vi "Switch.vi"(6 "Command Info In":T1, 8 "Position":T4=enum."Far Right") -> (0 "Command Info Out":T1)   [LabVIEW 2017]
uses:
  Support Code/Starting Position.ctl
  <vilib>/Rock Robotics/WPI/Framework/Command Status Info.ctl
  <vilib>/Rock Robotics/WPI/Framework/Completion Status.ctl
  <vilib>/Rock Robotics/WPI/Framework/Completion Notifier.ctl
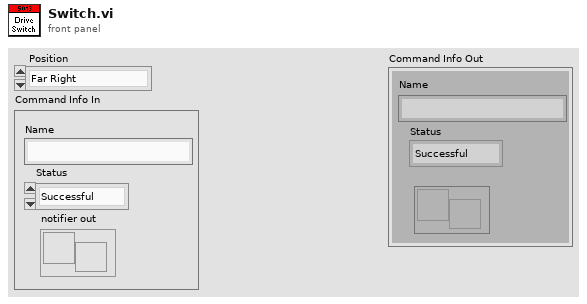
[diagram p1: front panel]
types:
  T1 = typedef "Command Status Info.ctl" = cluster{"Name":string, "Status":T2, "notifier out":T3}
  T2 = typedef "Completion Status.ctl" = enum16{"Successful", "Aborted", "Incomplete"}
  T3 = typedef "Completion Notifier.ctl" = refnum<notifier>
  T4 = typedef "Starting Position.ctl" = enum16{"Far Left", "Center", "Far Right"}
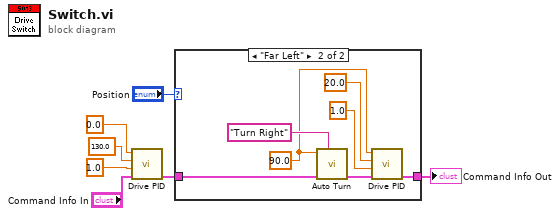
[diagram p0: block diagram]
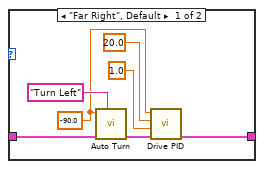
[diagram p2: hidden frame]
diagram:
  n1 = call "Drive PID.vi"("Command Info In"="Command Info In", "Speed"=1.0, "Distance"=130.0, "Target Angle"=0.0 ("Distance")) -> ("Command Info Out"=w5:T1)  [unwired: 7 in]
  n2 = case shown="\"Far Left\"" "Position" {
    tunnel: w5 -> [w14 w21]
    tunnel: [w8 w16] -> w2
    frame "Far Right", Default {
      w9 = -90.0 ("Target Angle")
      n3 = call "Auto Turn.vi"("Description"="Turn Left", "Command Info In"=w14, "Target Angle"=w9) -> ("Command Info Out"=w10:T1)  [unwired: 8 in]
      n4 = call "Drive PID.vi"("Command Info In"=w10, "Speed"=1.0, "Distance"=20.0, "Target Angle"=w9) -> ("Command Info Out"=w8:T1)  [unwired: 7 in]
    }
    frame "Far Left" {
      w15 = 90.0 ("Target Angle")
      n5 = call "Auto Turn.vi"("Description"="Turn Right", "Command Info In"=w21, "Target Angle"=w15) -> ("Command Info Out"=w17:T1)  [unwired: 8 in]
      n6 = call "Drive PID.vi"("Command Info In"=w17, "Speed"=1.0, "Distance"=20.0, "Target Angle"=w15) -> ("Command Info Out"=w16:T1)  [unwired: 7 in]
    }
  }
  "Command Info Out" <- w2
